vi "Program23.vi"() -> ()   [LabVIEW 2020]
uses:
  <vilib>/Utility/error.llb/DialogType.ctl
  <vilib>/Analysis/baseanly.llb/Mean (DBL).vi
  <vilib>/Utility/file.llb/Read Delimited Spreadsheet (DBL).vi
  <vilib>/Analysis/NI_AALBase.lvlib
  <vilib>/gmath/NI_Gmath.lvlib
panel:
  out "Q4":dbl[](array[numeric])
  out "Q3":dbl[](array[numeric])
  out "Q2":dbl[](array[numeric])
  out "Q1":dbl[](array[numeric])
  out "Calibration 3":path
  out "Calibration 2":path
  out "3.3Calibration loaded":bool
  out "3.2Calibration loaded":bool
  out "3.1Calibration loaded":bool
  in  "Manual":bool
  in  "REF3":dbl=1000.0 format="%#.0f"
  in  "REF2":dbl=1000.0 format="%#.0f"
  in  "REF1":dbl=1000.0 format="%#.0f"
  out "REF":dbl[](array[numeric])
  out "INT4":dbl[](array[numeric])
  out "S1+ S2 = Sx + Sy":bool
  out "Filenames":string[](array[string])
  out "INT3":dbl[](array[numeric])
  out "INT2":dbl[](array[numeric])
  out "INT1":dbl[](array[numeric])
  out "Wczytane":dbl[][](array[numeric])
  out "Loaded data":path
  out "Calibration":path
  out "Saved file":path
  in  "Save data":bool
  out "Beta":dbl[](array[numeric]) format="%#.0f"
  out "Sy":dbl[](array[numeric]) format="%#.0f"
  out "Sx":dbl[](array[numeric]) format="%#.0f"
  out "S2":dbl[](array[numeric]) format="%#.0f"
  out "S1":dbl[](array[numeric]) format="%#.0f"
  out "YY":dbl[][](array[numeric])
  out "XX":dbl[][](array[numeric])
  out "Data loaded":bool
  out "Calibration loaded":bool
  in  "0_45_90/45_90_135":bool
  in  "Run":bool
  in  "Stop":bool
  in  "Loda data":bool
  in  "Load calibration":bool
  in  "anisotropic?":bool
  in  "Poisson":dbl=0.33 min=0.0 max=1.0 step=0.01 format="%#_2g"
  in  "Young":dbl=0.22 min=0.0 max=1.0 step=0.01 format="%#_2g"
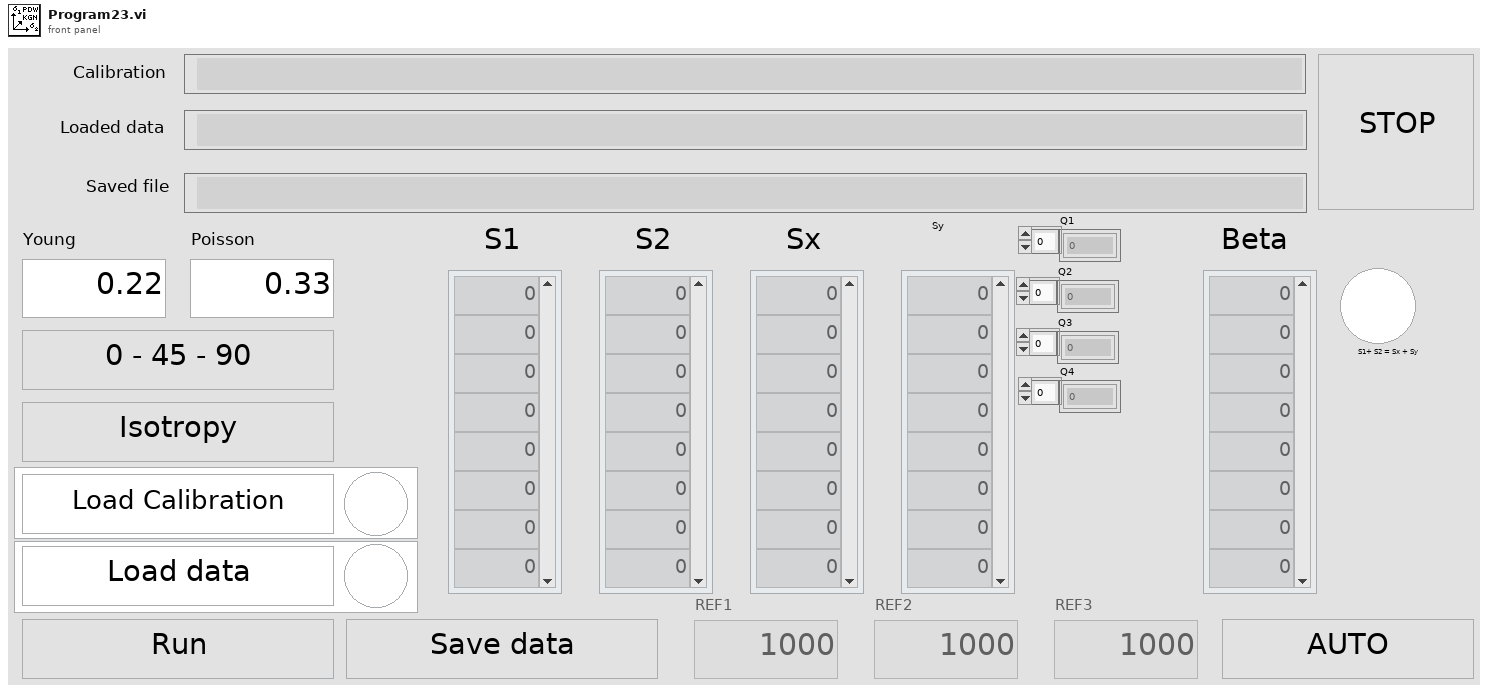
[diagram p1: front panel]
types:
  T1 = enum8{"Enabled", "Disabled", "Disabled and Grayed Out"}
  T2 = typedef "DialogType.ctl" = u16
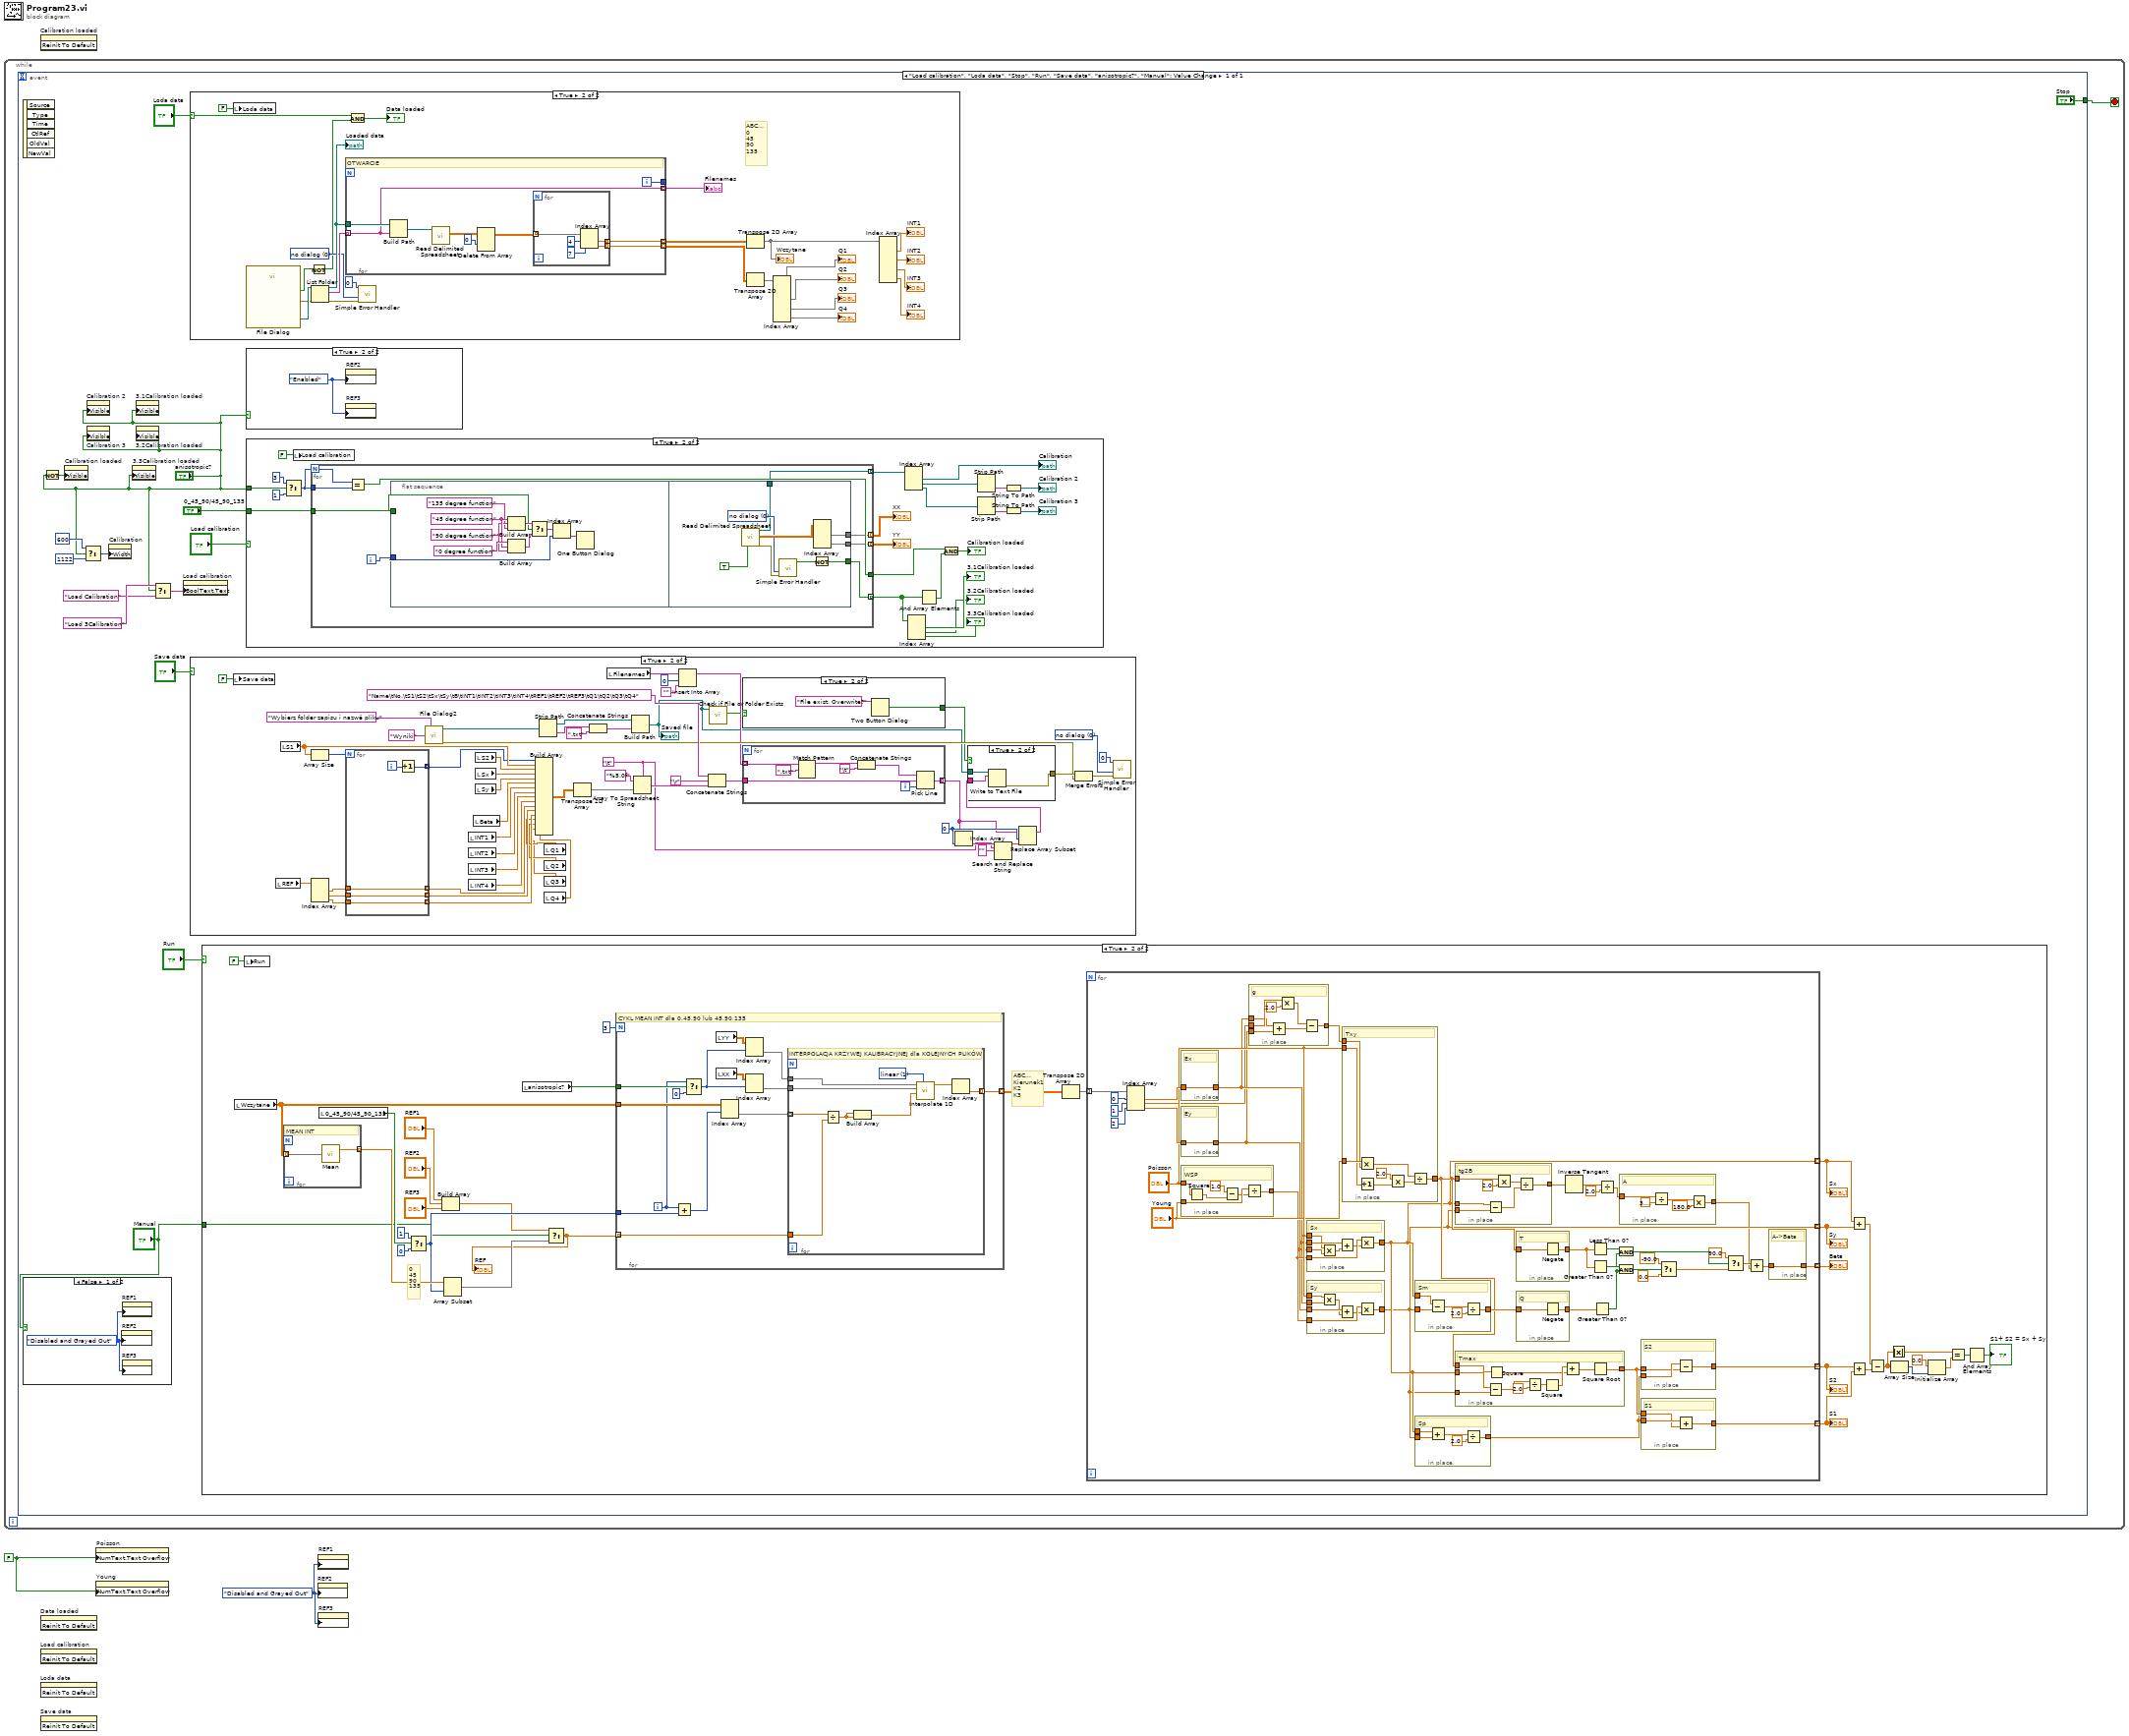
[diagram p0: block diagram]
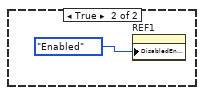
[diagram p2: hidden frame]
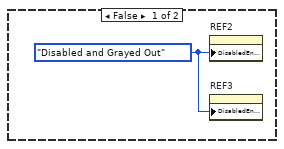
[diagram p3: hidden frame]
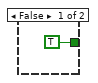
[diagram p5: hidden frame]
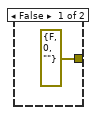
[diagram p6: hidden frame]
diagram:
  w1 = T1."Disabled and Grayed Out" ("Disabled")
  w2 = FALSE ("Numeric Text.Text Overflow")
  n1 = while {
    stop <- w3 stop-if-true
    n2 = event shown="[0] \"Load calibration\", \"Loda data\", \"Stop\", \"Run\", \"Save data\", \"anisotropic?\", \"Manual\": Value Change" {
      selector: _ -> [_]
      dyn-events: _ -> [_]
      timeout: _ -> [_]
      tunnel: ["Stop"] -> w3
      event "Load calibration", "Loda data", "Stop", "Run", "Save data", "anisotropic?", "Manual": Value Change {
        n3 = event-data() -> ()  [unwired: 1 in, 6 out]
        n4 = case shown="False" "Manual" {
          frame False {
            w19 = T1."Disabled and Grayed Out" ("Disabled")
            n5 = property on="REF2" class="DigNum (strict)"("DisabledEnum"=w19) -> ()  [unwired: 2 in, 2 out]
            n6 = property on="REF1" class="DigNum (strict)"("DisabledEnum"=w19) -> ()  [unwired: 2 in, 2 out]
            n7 = property on="REF3" class="DigNum (strict)"("DisabledEnum"=w19) -> ()  [unwired: 2 in, 2 out]
          }
          frame True {
            n8 = property on="REF1" class="DigNum (strict)"("DisabledEnum"=T1."Enabled" ("Disabled")) -> ()  [unwired: 2 in, 2 out]
          }
        }
        n9 = Not(x="anisotropic?") -> (.not. x?=w8:bool)
        n10 = property on="Calibration loaded" class="Bool (strict)"("Visible"=w8) -> ()  [unwired: 2 in, 2 out]
        n11 = Select(t=600, s="anisotropic?", f=1122) -> (s? t:f=w5:i32)
        n12 = property on="Calibration 2" class="Path"("Visible"="anisotropic?") -> ()  [unwired: 2 in, 2 out]
        n13 = property on="Calibration 3" class="Path"("Visible"="anisotropic?") -> ()  [unwired: 2 in, 2 out]
        n14 = property on="Calibration" class="Path"("Width"=w5) -> ()  [unwired: 2 in, 2 out]
        n15 = property on="3.3Calibration loaded" class="Bool (strict)"("Visible"="anisotropic?") -> ()  [unwired: 2 in, 2 out]
        n16 = property on="3.1Calibration loaded" class="Bool (strict)"("Visible"="anisotropic?") -> ()  [unwired: 2 in, 2 out]
        n17 = property on="3.2Calibration loaded" class="Bool (strict)"("Visible"="anisotropic?") -> ()  [unwired: 2 in, 2 out]
        n18 = Select(t="Load 3Calibration", s="anisotropic?", f="Load Calibration") -> (s? t:f=w11:string)
        n19 = property on="Load calibration" class="Bool (strict)"("BoolText.Text"=w11) -> ()  [unwired: 2 in, 2 out]
        n20 = case shown="True" "Loda data" {
          selector: "Loda data" -> [_ w291]
          frame False {
          }
          frame True {
            w292 = T2 0 items=["no dialog", "OK message", "continue or stop message", "OK message + warnings", "continue/stop + warnings"] ("type of dialog (OK msg:1)")
            # "ABC...\n0\n45\n90\n135"
            n21 = local write "Loda data"(FALSE ("Boolean")) -> ()
            n22 = call "File Dialog"() -> ("selected path"=w298:path, "cancelled"=w290:bool, "error out"=w294:errorcluster)  [unwired: 12 in, 1 out]
            n23 = Not(x=w290) -> (.not. x?=w289:bool)
            n24 = List Folder(path=w298, error in=w294) -> (path out=w299:path, filenames=w300:string[], error out=w293:errorcluster)  [unwired: 2 in, 1 out]
            "Loaded data" <- w299
            n25 = for {
              tunnel: w300 -> [w302] mode=indexing
              tunnel: w299 -> [w309]
              tunnel: [w304] -> w297 mode=indexing
              tunnel: [w303] -> _
              tunnel: [w302] -> w287 mode=indexing
              tunnel: [w301] -> w281 mode=indexing
              i -> [w303]
              # "OTWARCIE"
              n26 = Build Path(base path=w309, name or relative path=w302) -> (appended path=w308:path)
              n27 = call-poly <vilib>:"Read Delimited Spreadsheet.vi"("file path (dialog if empty)"=w308) -> ("all rows"=w307:dbl[][])  [unwired: 9 in, 5 out]
              n28 = Delete From Array(array=w307, index (row)=0) -> (array with subset deleted=w305:dbl[][])  [unwired: 2 in, 1 out]
              n29 = for {
                tunnel: w305 -> [w313] mode=indexing
                tunnel: [w312] -> w304 mode=indexing
                tunnel: [w310] -> w301 mode=indexing
                n30 = Index Array(array=w313, index #1=4 ("index"), index #2=7 ("index")) -> (element #1=w312:dbl, element #2=w310:dbl)
              }
            }
            "Filenames" <- w287
            n31 = And(x=w291, y=w289) -> (x .and. y?=→"Data loaded":bool)
            n32 = call <vilib>:"Simple Error Handler.vi"("error code (no error:0)"=0, "type of dialog (OK msg:1)"=w292, "error in (no error)"=w293) -> ()  [unwired: 2 in, 5 out]
            n33 = Transpose 2D Array(2D array=w297) -> (transposed array=w286:dbl[][])
            "Wczytane" <- w286
            n34 = Transpose 2D Array(2D array=w281) -> (transposed array=w280:dbl[][])
            n35 = Index Array(array=w280) -> (element #1=→"Q1":dbl[], element #2=→"Q2":dbl[], element #3=→"Q3":dbl[], element #4=→"Q4":dbl[])  [unwired: 8 in]
            n36 = Index Array(array=w286) -> (element #1=→"INT1":dbl[], element #2=→"INT2":dbl[], element #3=→"INT3":dbl[], element #4=→"INT4":dbl[])  [unwired: 8 in]
          }
        }
        n37 = case shown="True" "Save data" {
          frame False {
          }
          frame True {
            w33 = 0 ("index")
            w31 = "\t"
            w73 = T2 0 items=["no dialog", "OK message", "continue or stop message", "OK message + warnings", "continue/stop + warnings"] ("type of dialog (OK msg:1)")
            n38 = local write "Save data"(FALSE ("Save data")) -> ()
            n39 = local read "REF"() -> (w40:dbl[])
            n40 = local read "S1"() -> (w70:dbl[])
            n41 = Array Size(array=w70) -> (size(s)=w69:i32)
            n42 = Index Array(array=w40) -> (element #1=w39:dbl, element #2=w38:dbl, element #3=w37:dbl)  [unwired: 3 in]
            n43 = for {
              N: w69 -> [_]
              tunnel: [w97] -> w68 mode=indexing
              tunnel: w39 -> [w96]
              tunnel: w38 -> [w95]
              tunnel: w37 -> [w94]
              tunnel: [w96] -> w36 mode=indexing
              tunnel: [w95] -> w35 mode=indexing
              tunnel: [w94] -> w34 mode=indexing
              i -> [w98]
              n44 = Increment(x=w98) -> (x+1=w97:i32)
            }
            n45 = call "File Dialog2"("prompt"="Wybierz folder zapisu i nazwê pliku", "default name"="Wyniki") -> ("selected path"=w63:path, "error out"=w66:errorcluster)  [unwired: 10 in, 2 out]
            n46 = local read "INT1"() -> (w58:dbl[])
            n47 = local read "INT2"() -> (w57:dbl[])
            n48 = local read "INT3"() -> (w56:dbl[])
            n49 = local read "INT4"() -> (w41:dbl[])
            n50 = local read "Beta"() -> (w75:dbl[])
            n51 = local read "S2"() -> (w78:dbl[])
            n52 = local read "Sx"() -> (w77:dbl[])
            n53 = local read "Sy"() -> (w76:dbl[])
            n54 = Strip Path(path=w63) -> (stripped path=w62:path, name=w61:string)
            n55 = local read "Q1"() -> (w26:dbl[])
            n56 = local read "Q2"() -> (w25:dbl[])
            n57 = local read "Q3"() -> (w24:dbl[])
            n58 = local read "Q4"() -> (w23:dbl[])
            n59 = Build Array(w68, w70, w78, w77, w76, w75, w58, w57, w56, w41, w36, w35, w34, w26, w25, w24, w23) -> (w52:dbl[][])
            n60 = Transpose 2D Array(2D array=w52) -> (transposed array=w51:dbl[][])
            n61 = Concatenate Strings(w61, ".txt" ("string")) -> (w59:string)
            n62 = local read "Filenames"() -> (w49:string[])
            n63 = Build Path(base path=w62, name or relative path=w59) -> (appended path=w45:path)
            "Saved file" <- w45
            n64 = Array To Spreadsheet String(delimiter (Tab)=w31, array=w51, 3:"%5.0f" ("format string")) -> (spreadsheet string=w50:string)
            n65 = Insert Into Array(array=w49, index=0, new element="") -> (w46:string[])
            n66 = Concatenate Strings("Name\tNo.\tS1\tS2\tSx\tSy\tB\tINT1\tINT2\tINT3\tINT4\tREF1\tREF2\tREF3\tQ1\tQ2\tQ3\tQ4" ("string"), "\r", w50) -> (w53:string)
            n67 = call <vilib>:"Check if File or Folder Exists.vi"("path"=w45) -> ("file or folder exists?"=w43:bool)  [unwired: 8 in, 2 out]
            n68 = case shown="True" w43 {
              tunnel: [TRUE ("T button?") w80] -> w42
              frame False {
              }
              frame True {
                n69 = Two Button Dialog(message="File exist. Overwrite?") -> (T button?=w80:bool)  [unwired: 2 in]
              }
            }
            n70 = for {
              tunnel: w46 -> [w89] mode=indexing
              tunnel: w53 -> [w93]
              tunnel: [w92] -> w29 mode=indexing
              i -> [w90]
              n71 = Match Pattern(string=w89, regular expression=".txt") -> (before substring=w87:string)  [unwired: 1 in, 3 out]
              n72 = Concatenate Strings(w87, "\t") -> (w86:string)
              n73 = Pick Line(string ("")=w86, multi-line string=w93, line index=w90) -> (output string=w92:string)
            }
            n74 = Index Array(array=w29, index=w33) -> (element=w32:string)
            n75 = Search and Replace String(input string=w32, search string=w31, replace string="" ("replace string (\"\")")) -> (result string=w28:string)  [unwired: 5 in, 3 out]
            n76 = Replace Array Subset(array=w29, new element=w28, index=w33) -> (w27:string[])
            n77 = case shown="True" w42 {
              tunnel: [errorcluster {"status"=FALSE, "code"=0, "source"=""} ("error out") w85] -> w67
              tunnel: w27 -> [_ w84]
              tunnel: w45 -> [_ w83]
              frame False {
              }
              frame True {
                n78 = Write to Text File(file (use dialog)=w83, text=w84) -> (error out=w85:errorcluster)  [unwired: 2 in, 2 out]
              }
            }
            n79 = Merge Errors(w67, w66) -> (w65:errorcluster)
            n80 = call <vilib>:"Simple Error Handler.vi"("error code (no error:0)"=0, "type of dialog (OK msg:1)"=w73, "error in (no error)"=w65) -> ()  [unwired: 2 in, 5 out]
          }
        }
        n81 = case shown="True" "Run" {
          tunnel: "Manual" -> [_ w100]
          frame False {
          }
          frame True {
            # "ABC...\nKierunek1\nK2\nK3"
            # "0\n45\n90\n135"
            n82 = local read "Wczytane"() -> (w117:dbl[][])
            n83 = local write "Run"(FALSE ("Boolean")) -> ()
            n84 = for {
              tunnel: w117 -> [w155] mode=indexing
              tunnel: [w154] -> w116 mode=indexing
              # "MEAN INT"
              n85 = call-poly <vilib>:"Mean.vi"("X"=w155) -> ("mean"=w154:dbl)  [unwired: 1 out]
            }
            n86 = local read "0_45_90/45_90_135"() -> (w108:bool)
            n87 = Select(t=1, s=w108, f=0) -> (s? t:f=w109:i32)
            n88 = Build Array("REF1", "REF2", "REF3") -> (w102:dbl[])
            n89 = Array Subset(array=w116, index=w109) -> (w101:dbl[])  [unwired: 1 in]
            n90 = local read "anisotropic?"() -> (w107:bool)
            n91 = Select(t=w102, s=w100, f=w101) -> (s? t:f=w99:dbl[])
            "REF" <- w99
            n92 = for {
              N: 3 -> [_]
              tunnel: w99 -> [w144] mode=indexing
              tunnel: w117 -> [w141]
              tunnel: [w143] -> w112 mode=indexing
              tunnel: w109 -> [w136]
              tunnel: w107 -> [w134]
              i -> [w133]
              # "CYKL MEAN INT dla 0,45,90 lub 45,90,135"
              n93 = Add(x=w133, y=w136) -> (x+y=w135:i32)
              n94 = Select(t=w133, s=w134, f=0) -> (s? t:f=w132:i32)
              n95 = local read "YY"() -> (w139:dbl[][])
              n96 = local read "XX"() -> (w140:dbl[][])
              n97 = Index Array(array=w141, index (row)=w135) -> (element=w142:dbl[])  [unwired: 1 in]
              n98 = Index Array(array=w139, index (row)=w132) -> (element=w137:dbl[])  [unwired: 1 in]
              n99 = Index Array(array=w140, index (row)=w132) -> (element=w138:dbl[])  [unwired: 1 in]
              n100 = for {
                tunnel: w144 -> [w149]
                tunnel: [w147] -> w143 mode=indexing
                tunnel: w142 -> [w150] mode=indexing
                tunnel: w138 -> [w146]
                tunnel: w137 -> [w145]
                w153 = 1 items=["nearest", "linear", "spline", "cubic Hermite", "Lagrange"] ("method")
                # "INTERPOLACJA KRZYWEJ KALIBRACYJNEJ dla KOLEJNYCH PLIKÓW"
                n101 = Divide(x=w150, y=w149) -> (x/y=w152:dbl)
                n102 = Build Array(w152, w152) -> (w151:dbl[])
                n103 = call <vilib>:"Interpolate 1D.vi"("method"=w153, "xi"=w151, "X"=w146, "Y"=w145) -> ("yi"=w148:dbl[])  [unwired: 5 in, 2 out]
                n104 = Index Array(array=w148) -> (element=w147:dbl)  [unwired: 1 in]
              }
            }
            n105 = Transpose 2D Array(2D array=w112) -> (transposed array=w130:dbl[][])
            n106 = for {
              tunnel: [w195] -> w121 mode=indexing
              tunnel: [w194] -> w122 mode=indexing
              tunnel: w130 -> [w183] mode=indexing
              tunnel: [w178] -> w120 mode=indexing
              tunnel: [w179] -> w119 mode=indexing
              tunnel: [w166] -> w118 mode=indexing
              n107 = Index Array(array=w183, index #1=0 ("index"), index #2=1 ("index"), index #3=2 ("index")) -> (element #1=w191:dbl, element #2=w156:dbl, element #3=w192:dbl)
              n108 = in-place {
                in-place-border: w191 -> [w207]
                in-place-border: [w207] -> w158
                # "Ex"
              }
              n109 = in-place {
                in-place-border: w192 -> [w206]
                in-place-border: [w206] -> w157
                # "Ey"
              }
              n110 = in-place {
                in-place-border: "Young" -> [w253]
                in-place-border: "Poisson" -> [w251]
                in-place-border: [w248] -> w182
                # "WSP"
                n111 = Square(x=w251) -> (x^2=w250:dbl)
                n112 = Subtract(x=1.0, y=w250) -> (x-y=w249:dbl)
                n113 = Divide(x=w253, y=w249) -> (x/y=w248:dbl)
              }
              n114 = in-place {
                in-place-border: w156 -> [w260]
                in-place-border: w158 -> [w258]
                in-place-border: w157 -> [w257]
                in-place-border: [w254] -> w181
                # "g"
                n115 = Add(x=w258, y=w257) -> (x+y=w255:dbl)
                n116 = Multiply(x=w260, y=2.0) -> (x*y=w256:dbl)
                n117 = Subtract(x=w256, y=w255) -> (x-y=w254:dbl)
              }
              n118 = in-place {
                in-place-border: w182 -> [w267]
                in-place-border: w158 -> [w266]
                in-place-border: "Poisson" -> [w265]
                in-place-border: w157 -> [w264]
                in-place-border: [w261] -> w179
                # "Sx"
                n119 = Multiply(x=w265, y=w264) -> (x*y=w263:dbl)
                n120 = Add(x=w266, y=w263) -> (x+y=w262:dbl)
                n121 = Multiply(x=w267, y=w262) -> (x*y=w261:dbl)
              }
              n122 = in-place {
                in-place-border: w182 -> [w247]
                in-place-border: w157 -> [w246]
                in-place-border: "Poisson" -> [w245]
                in-place-border: w158 -> [w244]
                in-place-border: [w241] -> w178
                # "Sy"
                n123 = Multiply(x=w245, y=w244) -> (x*y=w243:dbl)
                n124 = Add(x=w246, y=w243) -> (x+y=w242:dbl)
                n125 = Multiply(x=w247, y=w242) -> (x*y=w241:dbl)
              }
              n126 = in-place {
                in-place-border: "Young" -> [w275]
                in-place-border: w181 -> [w274]
                in-place-border: "Poisson" -> [w269]
                in-place-border: [w268] -> w180
                # "Txy"
                n127 = Multiply(x=w275, y=w274) -> (x*y=w273:dbl)
                n128 = Increment(x=w269) -> (x+1=w270:dbl)
                n129 = Multiply(x=2.0, y=w270) -> (x*y=w272:dbl)
                n130 = Divide(x=w273, y=w272) -> (x/y=w268:dbl)
              }
              n131 = in-place {
                in-place-border: w179 -> [w235]
                in-place-border: w178 -> [w234]
                in-place-border: [w231] -> w193
                # "Sm"
                n132 = Subtract(x=w235, y=w234) -> (x-y=w232:dbl)
                n133 = Divide(x=w232, y=2.0) -> (x/y=w231:dbl)
              }
              n134 = in-place {
                in-place-border: w179 -> [w240]
                in-place-border: w178 -> [w239]
                in-place-border: [w236] -> w189
                # "Sp"
                n135 = Add(x=w240, y=w239) -> (x+y=w237:dbl)
                n136 = Divide(x=w237, y=2.0) -> (x/y=w236:dbl)
              }
              n137 = in-place {
                in-place-border: w180 -> [w213]
                in-place-border: w179 -> [w211]
                in-place-border: w178 -> [w210]
                in-place-border: [w208] -> w165
                # "tg2B"
                n138 = Subtract(x=w211, y=w210) -> (x-y=w209:dbl)
                n139 = Multiply(x=w213, y=2.0) -> (x*y=w212:dbl)
                n140 = Divide(x=w212, y=w209) -> (x/y=w208:dbl)
              }
              n141 = in-place {
                in-place-border: w179 -> [w224]
                in-place-border: w178 -> [w223]
                in-place-border: w180 -> [w222]
                in-place-border: [w221] -> w190
                # "Tmax"
                n142 = Subtract(x=w224, y=w223) -> (x-y=w227:dbl)
                n143 = Square(x=w222) -> (x^2=w228:dbl)
                n144 = Divide(x=w227, y=2.0) -> (x/y=w225:dbl)
                n145 = Square(x=w225) -> (x^2=w229:dbl)
                n146 = Add(x=w229, y=w228) -> (x+y=w230:dbl)
                n147 = Square Root(x=w230) -> (sqrt(x)=w221:dbl)
              }
              n148 = in-place {
                in-place-border: w180 -> [w203]
                in-place-border: [w202] -> w177
                # "T"
                n149 = Negate(x=w203) -> (-x=w202:dbl)
              }
              n150 = in-place {
                in-place-border: w193 -> [w205]
                in-place-border: [w204] -> w176
                # "Q"
                n151 = Negate(x=w205) -> (-x=w204:dbl)
              }
              n152 = Inverse Tangent(1:w165) -> (0:w163:dbl)
              n153 = Less Than 0?(x=w177) -> (x < 0?=w170:bool)
              n154 = Greater Than 0?(x=w177) -> (x > 0?=w175:bool)
              n155 = Greater Than 0?(x=w176) -> (x > 0?=w171:bool)
              n156 = Divide(x=w163, y=2.0) -> (x/y=w162:dbl)
              n157 = And(x=w170, y=w171) -> (x .and. y?=w169:bool)
              n158 = And(x=w175, y=w171) -> (x .and. y?=w173:bool)
              n159 = in-place {
                in-place-border: w162 -> [w200]
                in-place-border: [w196] -> w159
                # "A"
                n160 = Divide(x=w200, y=3.141592653589793) -> (x/y=w198:dbl)
                n161 = Multiply(x=w198, y=180.0) -> (x*y=w196:dbl)
              }
              n162 = in-place {
                in-place-border: w189 -> [w217]
                in-place-border: w190 -> [w216]
                in-place-border: [w215] -> w195
                # "S2"
                n163 = Subtract(x=w217, y=w216) -> (x-y=w215:dbl)
              }
              n164 = in-place {
                in-place-border: w189 -> [w220]
                in-place-border: w190 -> [w219]
                in-place-border: [w218] -> w194
                # "S1"
                n165 = Add(x=w220, y=w219) -> (x+y=w218:dbl)
              }
              n166 = Select(t=-90.0, s=w173, f=0.0) -> (s? t:f=w168:dbl)
              n167 = Select(t=90.0, s=w169, f=w168) -> (s? t:f=w161:dbl)
              n168 = Add(x=w161, y=w159) -> (x+y=w160:dbl)
              n169 = in-place {
                in-place-border: w160 -> [w201]
                in-place-border: [w201] -> w166
                # "A->Beta"
              }
            }
            "S1" <- w122
            "Beta" <- w118
            "Sy" <- w120
            "S2" <- w121
            "Sx" <- w119
            n170 = Add(x=w119, y=w120) -> (x+y=w129:dbl[])
            n171 = Add(x=w121, y=w122) -> (x+y=w128:dbl[])
            n172 = Subtract(x=w129, y=w128) -> (x-y=w127:dbl[])
            n173 = Absolute Value(x=w127) -> (abs(x)=w124:dbl[])
            n174 = Array Size(array=w127) -> (size(s)=w125:i32)
            n175 = Initialize Array(0.0 ("element"), w125) -> (w123:dbl[])
            n176 = Equal?(x=w124, y=w123) -> (x = y?=w111:bool[])
            n177 = And Array Elements(Boolean array=w111) -> (logical AND=→"S1+ S2 = Sx + Sy":bool)
          }
        }
        n178 = case shown="True" "anisotropic?" {
          frame False {
            w21 = T1."Disabled and Grayed Out" ("Disabled")
            n179 = property on="REF2" class="DigNum (strict)"("DisabledEnum"=w21) -> ()  [unwired: 2 in, 2 out]
            n180 = property on="REF3" class="DigNum (strict)"("DisabledEnum"=w21) -> ()  [unwired: 2 in, 2 out]
          }
          frame True {
            w22 = T1."Enabled" ("Disabled")
            n181 = property on="REF2" class="DigNum (strict)"("DisabledEnum"=w22) -> ()  [unwired: 2 in, 2 out]
            n182 = property on="REF3" class="DigNum (strict)"("DisabledEnum"=w22) -> ()  [unwired: 2 in, 2 out]
          }
        }
        n183 = case shown="True" "Load calibration" {
          tunnel: "anisotropic?" -> [_ w328]
          tunnel: "0_45_90/45_90_135" -> [_ w327]
          frame False {
          }
          frame True {
            n184 = Select(t=3, s=w328, f=1) -> (s? t:f=w331:i32)
            n185 = local write "Load calibration"(FALSE ("Load calibration")) -> ()
            n186 = for {
              N: w331 -> [w342]
              tunnel: w327 -> [w345]
              tunnel: [w344] -> w326 mode=indexing
              tunnel: [w343] -> w333
              tunnel: w331 -> [w341]
              tunnel: [w340] -> w330 mode=indexing
              tunnel: [w339] -> w329 mode=indexing
              tunnel: [w338] -> w322 mode=indexing
              i -> [w346]
              n187 = Equal?(x=w342, y=w341) -> (x = y?=w343:bool)
              n188 = flat-sequence {
                tunnel: w346 -> [w347]
                tunnel: w345 -> [w349]
                tunnel: [w360] -> w344
                tunnel: [w359] -> w340
                tunnel: [w358] -> w339
                tunnel: [w357] -> w338
                frame #0 {
                  w353 = "90 degree function"
                  w354 = "45 degree function"
                  n189 = Build Array(w354, w353, "135 degree function") -> (w351:string[])
                  n190 = Build Array("0 degree function", w354, w353) -> (w350:string[])
                  n191 = Select(t=w351, s=w349, f=w350) -> (s? t:f=w348:string[])
                  n192 = Index Array(array=w348, index=w347) -> (element=w355:string)
                  n193 = One Button Dialog(message=w355) -> ()  [unwired: 1 in, 1 out]
                }
                frame #1 {
                  w363 = T2 0 items=["no dialog", "OK message", "continue or stop message", "OK message + warnings", "continue/stop + warnings"] ("type of dialog (OK msg:1)")
                  n194 = call-poly <vilib>:"Read Delimited Spreadsheet.vi"("transpose? (F)"=TRUE) -> ("new file path (Not A Path if cancelled)"=w357:path, "all rows"=w364:dbl[][], "error out"=w365:errorcluster)  [unwired: 9 in, 3 out]
                  n195 = call <vilib>:"Simple Error Handler.vi"("type of dialog (OK msg:1)"=w363, "error in (no error)"=w365) -> ("error?"=w361:bool)  [unwired: 3 in, 4 out]
                  n196 = Not(x=w361) -> (.not. x?=w360:bool)
                  n197 = Index Array(array=w364) -> (element #1=w359:dbl[], element #2=w358:dbl[])  [unwired: 4 in]
                }
              }
            }
            "XX" <- w330
            "YY" <- w329
            n198 = Index Array(array=w322) -> (element #1=→"Calibration":path, element #2=w318:path, element #3=w317:path)  [unwired: 3 in]
            n199 = Index Array(array=w326) -> (element #1=→"3.1Calibration loaded":bool, element #2=→"3.2Calibration loaded":bool, element #3=→"3.3Calibration loaded":bool)  [unwired: 3 in]
            n200 = And Array Elements(Boolean array=w326) -> (logical AND=w334:bool)
            n201 = And(x=w333, y=w334) -> (x .and. y?=→"Calibration loaded":bool)
            n202 = Strip Path(path=w318) -> (name=w315:string)  [unwired: 1 out]
            n203 = Strip Path(path=w317) -> (name=w316:string)  [unwired: 1 out]
            n204 = String To Path(string=w315) -> (path=→"Calibration 2":path)
            n205 = String To Path(string=w316) -> (path=→"Calibration 3":path)
          }
        }
      }
    }
  }
  n206 = invoke on="Calibration loaded" class="Bool (strict)" method="Reinit To Default"() -> ()  [unwired: 3 in, 3 out]
  n207 = invoke on="Data loaded" class="Bool (strict)" method="Reinit To Default"() -> ()  [unwired: 3 in, 3 out]
  n208 = invoke on="Load calibration" class="Bool (strict)" method="Reinit To Default"() -> ()  [unwired: 3 in, 3 out]
  n209 = invoke on="Loda data" class="Bool (strict)" method="Reinit To Default"() -> ()  [unwired: 3 in, 3 out]
  n210 = invoke on="Save data" class="Bool (strict)" method="Reinit To Default"() -> ()  [unwired: 3 in, 3 out]
  n211 = property on="Poisson" class="DigNum (strict)"("NumText.Text Overflow"=w2) -> ()  [unwired: 2 in, 2 out]
  n212 = property on="Young" class="DigNum (strict)"("NumText.Text Overflow"=w2) -> ()  [unwired: 2 in, 2 out]
  n213 = property on="REF2" class="DigNum (strict)"("DisabledEnum"=w1) -> ()  [unwired: 2 in, 2 out]
  n214 = property on="REF1" class="DigNum (strict)"("DisabledEnum"=w1) -> ()  [unwired: 2 in, 2 out]
  n215 = property on="REF3" class="DigNum (strict)"("DisabledEnum"=w1) -> ()  [unwired: 2 in, 2 out]
